vi "Handle Remote Command.vi"(8 "error in (no error)":errorcluster, 9 "Data":string, 10 "Command":string, 11 "Instrument in":refnum<class "Instrument.lvclass">) -> (0 "error out":errorcluster, 2 "Variant":variant, 3 "Instrument out":refnum<class "Instrument.lvclass">)   [LabVIEW 2016, in "Instrument.lvclass"]
uses:
  Instrument.lvclass
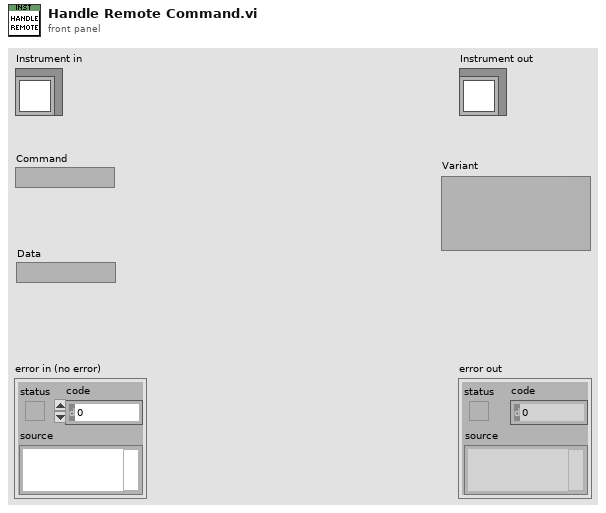
[diagram p1: front panel]
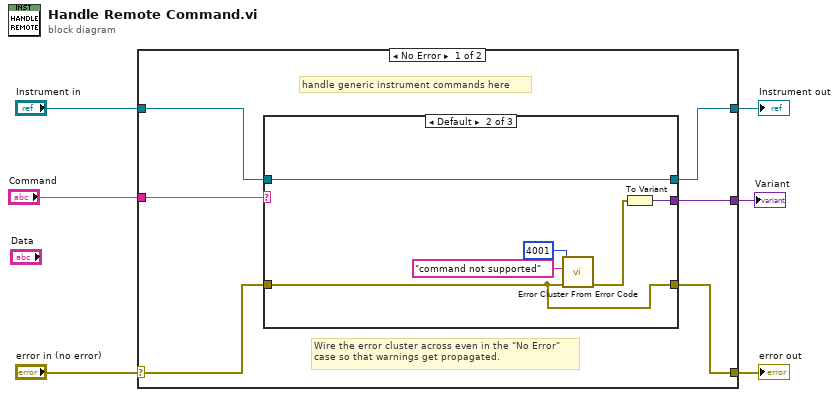
[diagram p0: block diagram]
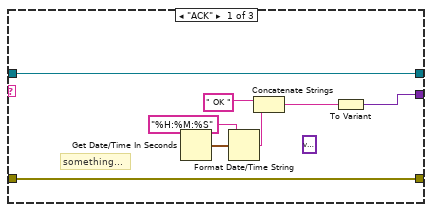
[diagram p2: hidden frame]
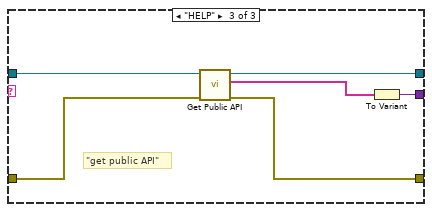
[diagram p3: hidden frame]
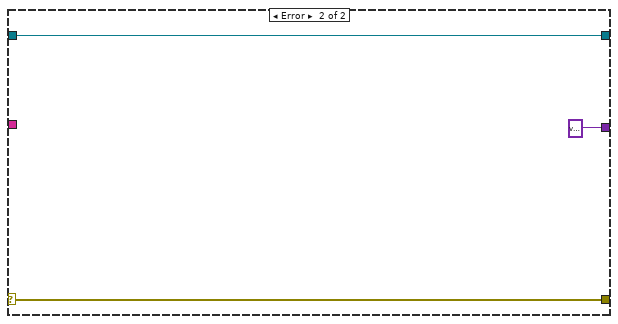
[diagram p4: hidden frame]
diagram:
  n1 = case shown="No Error" "error in (no error)" {
    selector: "error in (no error)" -> [w8 w35]
    tunnel: [w7 w35] -> w5
    tunnel: [w10 w34] -> w3
    tunnel: "Instrument in" -> [w11 w34]
    tunnel: "Command" -> [w12 _]
    tunnel: [w9 variant ("Variant")] -> w1
    frame No Error {
      # "handle generic instrument commands here"
      # "Wire the error cluster across even in the \"No Error\"\ncase so that warnings get propagated."
      n2 = case shown="Default" w12 {
        tunnel: w11 -> [w20 w24 w32]
        tunnel: [w20 w24 w31] -> w10
        tunnel: [w13 w22 w28] -> w9
        tunnel: w8 -> [w19 w23 w29]
        tunnel: [w19 w23 w30] -> w7
        frame "ACK" {
          (unwired) variant ("Variant")
          # "something..."
          n3 = Get Date/Time In Seconds() -> (seconds since 1Jan1904=w16:timestamp)
          n4 = Format Date/Time String(time format string (%c)="%H:%M:%S", seconds (now)=w16) -> (date/time string=w17:string)  [unwired: 1 in]
          n5 = Concatenate Strings(" OK " ("data"), w17) -> (w14:string)
          n6 = To Variant(anything=w14) -> (Variant=w13:variant)
        }
        frame Default {
          n7 = call <vilib>:"Error Cluster From Error Code.vi"("error in (no error)"=w23, "error message (\"\")"="command not supported" ("error message (\"\")"), "error code (0)"=4001) -> ("error out"=w21:errorcluster)  [unwired: 6 in]
          n8 = To Variant(anything=w21) -> (Variant=w22:variant)
        }
        frame "HELP" {
          # "\"get public API\""
          n9 = call-dynamic "Get Public API.vi"("error in (no error)"=w29, "Instrument in"=w32) -> ("error out"=w30:errorcluster, "Array"=w27:string[], "Instrument out"=w31:refnum<class "Instrument.lvclass">)  [unwired: 7 in]
          n10 = To Variant(anything=w27) -> (Variant=w28:variant)
        }
      }
    }
    frame Error {
    }
  }
  "error out" <- w5
  "Instrument out" <- w3
  "Variant" <- w1
